vi "Construct Wait forTransfer State.vi"(7 "Array of States to wait for":T1[](array[typedef]), 8 "error in (no error)":errorcluster, 9 "Timeout (5 sec)":dbl=5.0 caption="Time Target (s)") -> (0 "error out":errorcluster, 1 "Timed out?":bool)   [LabVIEW 2015]
uses:
  Controls/Sample Transfer State Enumerator.ctl
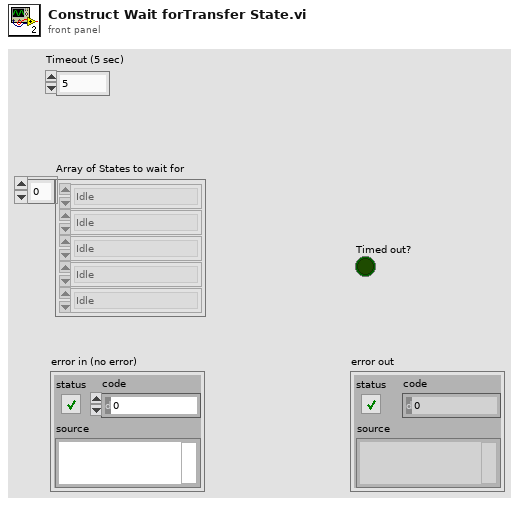
[diagram p1: front panel]
types:
  T1 = typedef "Sample Transfer State Enumerator.ctl" = enum16{"Idle", "Initialize", "Check Containers", "Check Temperatures", "Start Turbo", "Warm Up Containers", "Prepare for purging", "Purge Capillary", "Purge", "Open Containers", "Introduce Sample", "Measure Base Pressure", "Home Syringe", "Start Freezer", "Freeze Target", "Crystalize", "Stash", "Polish", "Stop Freezers", "Push Sample", "Complete", "Abort", "Error", "Undefined"}
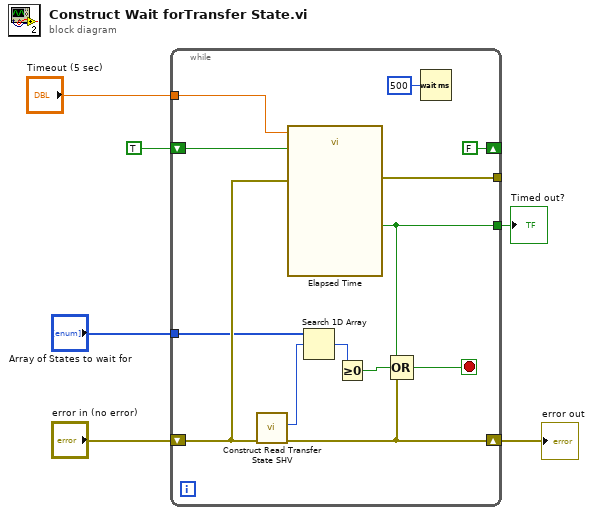
[diagram p0: block diagram]
diagram:
  n1 = while {
    tunnel: "Array of States to wait for" -> [w10]
    shift-right: [w18] -> w5
    shift-left: "error in (no error)" -> [w14]
    shift-right: [FALSE] -> _
    shift-left: TRUE -> [w17]
    tunnel: "Timeout (5 sec)" -> [w15]
    tunnel: [w13] -> _
    tunnel: [w12] -> w1
    stop <- w19 stop-if-true
    n2 = call "Construct Read Transfer State SHV.vi"("error in (no error)"=w14) -> ("error out"=w18:errorcluster, "State"=w9:T1)  [unwired: 9 in]
    n3 = call "Elapsed Time"("Time Target (s)"=w15, "Reset"=w17, "error in (no error)"=w14) -> ("Time has Elapsed"=w12:bool, "error out"=w13:errorcluster)  [unwired: 9 in, 6 out]
    n4 = Search 1D Array(1D array=w10, element=w9) -> (index of element=w8:i32)  [unwired: 1 in]
    n5 = Greater Or Equal To 0?(x=w8) -> (x >= 0?=w7:bool)
    n6 = Compound Arithmetic op=OR(w12, w7, w18) -> (w19:bool)
    n7 = Wait (ms)(milliseconds to wait=u32 500) -> ()  [unwired: 1 out]
  }
  "error out" <- w5
  "Timed out?" <- w1
